vi "未命名 5.vi"   [LabVIEW 2011]
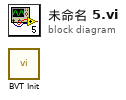
[diagram p0: block diagram]
diagram:
  n1 = call <userlib>:"BVT Init.vi"() -> ()  [unwired: 11 in, 1 out]
